vi "Unflatten from String.vi"(8 "error in (no error)":errorcluster, 10 "Flattened String":string, 11 "Serializable Flattener in":refnum<class "Serializable Flattener.lvclass">) -> (0 "error out":errorcluster, 1 "priority":i32, 2 "Message":refnum<class "Message.lvclass">, 3 "Serializable Flattener out":refnum<class "Serializable Flattener.lvclass">)   [LabVIEW 2020, in "Serializer.lvlib" / "Serializable Flattener.lvclass"]
uses:
  Serializable Flattener.lvclass
  <vilib>/ActorFramework/Message/Message.lvclass
  Cache Manager/Cache Manager.lvclass/Cache Manager.ctl
  Cache Manager/accessors/Get Object by Class name new.vi
  Serializable Message/Serializable Msg.lvclass
  C:/Program Files (x86)/National Instruments/LabVIEW 2020/vi.lib/ActorFramework/Message/Message.lvclass
  <vilib>/Utility/LVClass/Get LV Class Default Value By Name.vi
  Serializable Flattener.lvclass/Serializable Flattener.ctl
  Cache Manager/Cache Manager.lvclass
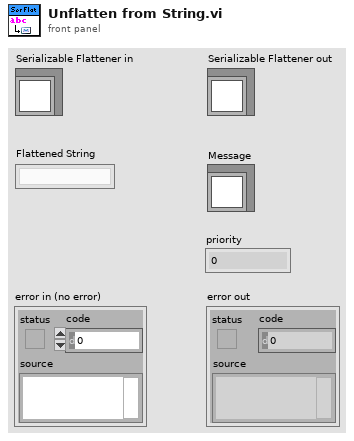
[diagram p1: front panel]
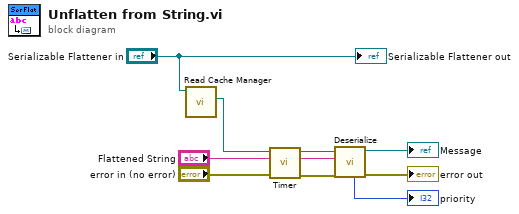
[diagram p0: block diagram]
diagram:
  n1 = call-dynamic "Read Cache Manager.vi"("Message Flattener in"="Serializable Flattener in") -> ("Cache Manager DVR.lvclass"=w4:refnum<class "Cache Manager.lvclass">)  [unwired: 9 in, 1 out]
  n2 = call "Timer.vi"("error in (no error)"="error in (no error)", "Cache Manager DVR in"=w4) -> ("error out"=w1:errorcluster, "Cache Manager DVR out"=w3:refnum<class "Cache Manager.lvclass">)  [unwired: 7 in, 1 out]
  n3 = call "Deserialize.vi"("error in (no error)"=w1, "Serialized Message"="Flattened String", "Cache Manager DVR"=w3) -> ("error out"=→"error out":errorcluster, "Serialize out"=→"Message":refnum<class "Serializable Msg.lvclass">, "priority"=→"priority":i32)  [unwired: 6 in]
  "Serializable Flattener out" <- "Serializable Flattener in"
